vi "Exit For Loop.vi"(0 "Diagram in":refnum<vi>, 1 "Conditional Terminals":refnum<vi>[](array[refnum]), 2 "Loop Terminal Types":T1[](array[typedef]), 5 "Outputs":refnum<vi>[](array[refnum]), 7 "Shift Registers":refnum<vi>[](array[refnum]), 9 "Stop Condition":refnum<vi>, 11 "error in (no error)":errorcluster) -> (4 "Diagram out":refnum<vi>, 6 "Outputs":refnum<vi>[](array[refnum]), 8 "Shift Registers":refnum<vi>[](array[refnum]), 15 "error out":errorcluster)   [LabVIEW 2015, in "Scripting.lvlib"]
doc: "Exits the For Loop that owns <B>Diagram in</B>, supplying the structure's owning diagram at <B>Diagram out</B>.\n\n<B>Stop Condition</B> is optionally the terminal to wire to the conditional terminal of the For Loop.\n\n<B>Conditional Terminals</B> is optionally an array of terminals to wire to the conditional terminal of the For Loop's output tunnels.\n\n<B>Loop Terminal Types</B> is optionally and array of terminal types of the For Loop's output tunnels."
uses:
  Scripting.lvlib
  Loop Terminal Type.ctl
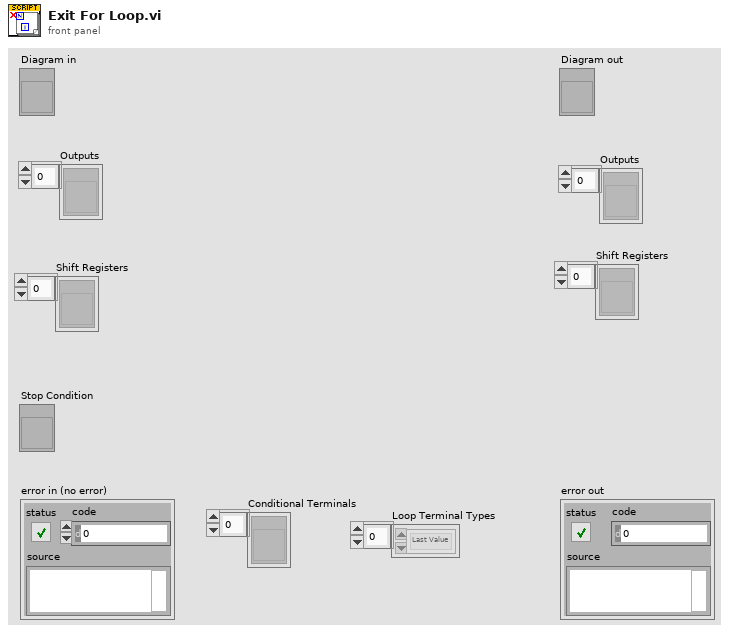
[diagram p1: front panel]
types:
  T1 = typedef "Scripting.lvlib/Loop Terminal Type.ctl" = enum16{"Last Value", "Indexing", "Concatenating"}
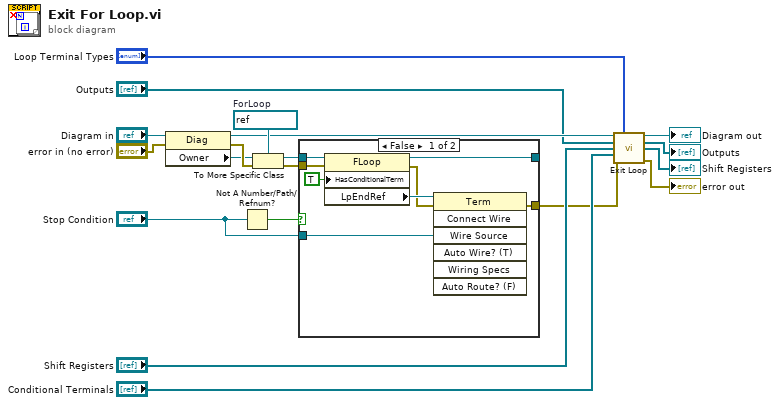
[diagram p0: block diagram]
diagram:
  w18 = refnum<vi> refnum  # ForLoop
  n1 = property class="Diag"(reference="Diagram in", error in="error in (no error)") -> (reference out=w14:refnum<vi>, error out=w19:errorcluster, "Owner"=w17:refnum<vi>)
  n2 = Not A Number/Path/Refnum?(number/path/refnum="Stop Condition") -> (NaN/Path/Refnum?=w11:bool)
  n3 = To More Specific Class(target class=w18, reference=w17, error in=w19) -> (specific class reference=w7:refnum<vi>, error out=w6:errorcluster)
  n4 = case shown="False" w11 {
    tunnel: "Stop Condition" -> [w27 _]
    tunnel: [w26 w29] -> w3
    tunnel: w7 -> [w25 w28]
    tunnel: w6 -> [w24 w29]
    tunnel: [w20 w28] -> _
    frame False {
      n5 = property class="FLoop"(reference=w25, error in=w24, "HasConditionalTerm"=TRUE ("Has Conditional Terminal?")) -> (reference out=w20:refnum<vi>, error out=w21:errorcluster, "LpEndRef"=w22:refnum<vi>)
      n6 = invoke class="Term" method="Connect Wire"(reference=w22, error in=w21, "Wire Source"=w27) -> (error out=w26:errorcluster)  [unwired: 4 in, 6 out]
    }
    frame True {
    }
  }
  n7 = call "Exit Loop.vi"("Diagram in"=w14, "Loop Terminal Types"="Loop Terminal Types", "Outputs"="Outputs", "Shift Registers"="Shift Registers", "Conditional Terminals"="Conditional Terminals", "error in (no error)"=w3) -> ("Diagram out"=→"Diagram out":refnum<vi>, "Outputs"=→"Outputs":refnum<vi>[], "Shift Registers"=→"Shift Registers":refnum<vi>[], "error out"=→"error out":errorcluster)  [unwired: 6 in]
